vi "debug.vi"() -> ()   [LabVIEW 2020]
uses:
  Test Finder.lvclass
panel:
  in  "Class Ancestry 2":path[](array[path])
  out "Class Ancestry":path[][](array[path])
  out "Array 2":string[](array[string])
  out "Array":path[](array[path])
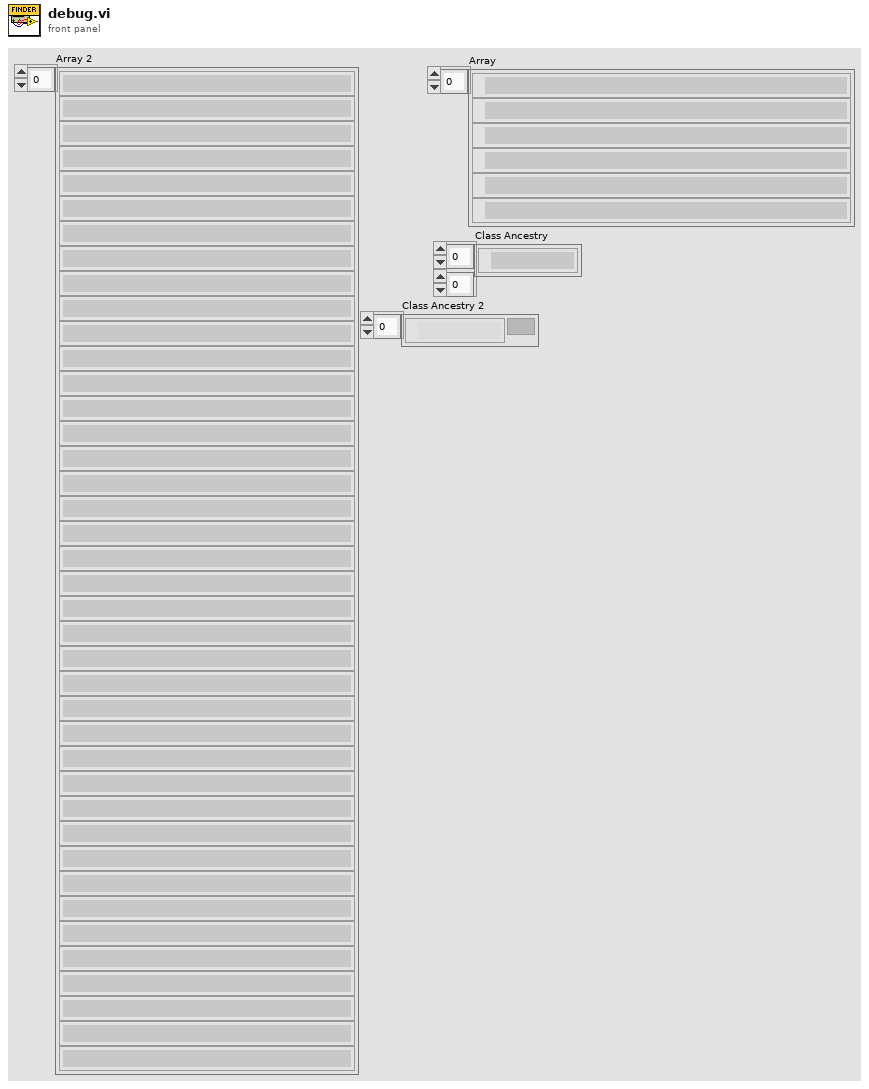
[diagram p1: front panel]
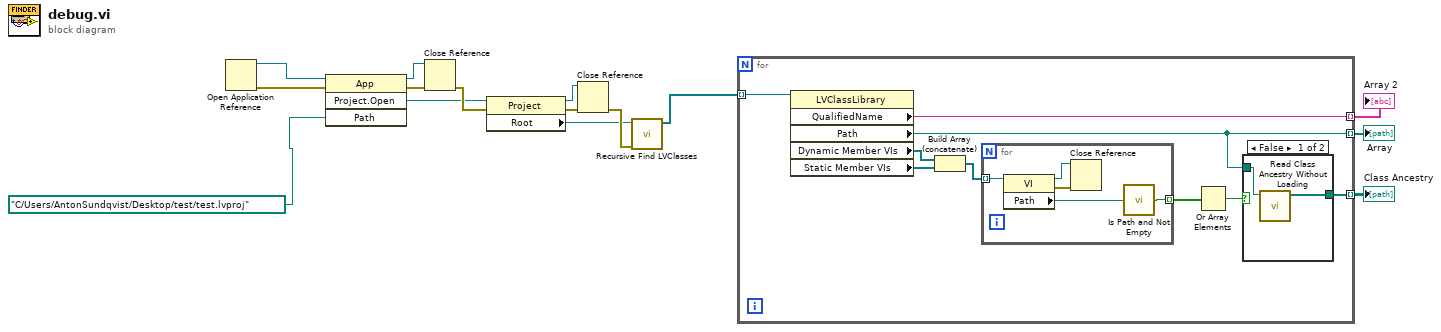
[diagram p0: block diagram]
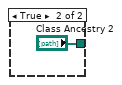
[diagram p2: hidden frame]
diagram:
  n1 = Open Application Reference() -> (0:w9:errorcluster, 3:w8:refnum<vi>)  [unwired: 4 in]
  n2 = invoke class="App" method="Project.Open"(reference=w8, error in=w9, "Path"=path "C:/Users/AntonSundqvist/Desktop/test/test.lvproj") -> (reference out=w11:refnum<vi>, error out=w10:errorcluster, "Project:Open"=w1:refnum<vi>)  [unwired: 1 in, 1 out]
  n3 = Close Reference(reference=w11, error in (no error)=w10) -> (error out=w12:errorcluster)
  n4 = property class="Project"(reference=w1, error in=w12) -> (reference out=w15:refnum<vi>, error out=w13:errorcluster, "Root"=w7:refnum<vi>)
  n5 = Close Reference(reference=w15, error in (no error)=w13) -> (error out=w14:errorcluster)
  n6 = call "Recursive Find LVClasses.vi"("error in (no error)"=w14, "reference"=w7) -> ("Class References"=w6:refnum<vi>[])  [unwired: 8 in, 1 out]
  n7 = for {
    tunnel: [w24] -> w4 mode=indexing
    tunnel: [w22] -> w5 mode=indexing
    tunnel: w6 -> [w23] mode=indexing
    tunnel: [w21] -> w2 mode=indexing
    n8 = property class="LVClassLibrary"(reference=w23) -> ("QualifiedName"=w24:string, "Path"=w22:path, "Dynamic Member VIs"=w20:refnum<vi>[], "Static Member VIs"=w19:refnum<vi>[])  [unwired: 1 in, 2 out]
    n9 = Build Array (concatenate)(w20, w19) -> (w18:refnum<vi>[])
    n10 = for {
      tunnel: w18 -> [w32] mode=indexing
      tunnel: [w30] -> w17 mode=indexing
      n11 = property class="VI"(reference=w32) -> (reference out=w28:refnum<vi>, error out=w29:errorcluster, "Path"=w31:path)  [unwired: 1 in]
      n12 = Close Reference(reference=w28, error in (no error)=w29) -> ()  [unwired: 1 out]
      n13 = call <vilib>:"Is Path and Not Empty.vi"("path"=w31) -> ("Is Path and Not Empty?"=w30:bool)  [unwired: 4 in]
    }
    n14 = Or Array Elements(Boolean array=w17) -> (logical OR=w16:bool)
    n15 = case shown="False" w16 {
      tunnel: w22 -> [w26 _]
      tunnel: [w25 "Class Ancestry 2"] -> w21
      frame False {
        n16 = call <vilib>:"Read Class Ancestry Without Loading.vi"("LabVIEW Class Path"=w26) -> ("Class Ancestry"=w25:path[])  [unwired: 9 in, 1 out]
      }
      frame True {
      }
    }
  }
  "Array" <- w5
  "Array 2" <- w4
  "Class Ancestry" <- w2
